vi "Get All Measured Values.vi"(0 "VISA Session In":refnum<visa-resource-name>="OXYMAT", 1 "Target Address":u8=16 format="%.0x", 2 "Source Address":u8=208 format="%.0x", 7 "Use Broadcast?(F)":bool, 11 "error in (no error)":errorcluster) -> (4 "VISA Session Out":refnum<visa-resource-name>, 6 "Message Header":T3 {"Source Address" format="%.0x"; "Target Address" format="%.0x"}, 8 "Measurements":cluster{"Measured value":dbl, "Dimension":T1}[](array[cluster]) {"Measured value" format="%#_6f"}, 10 "Measured variables":T2[](array[typedef]), 13 "Success":bool, 15 "error out":errorcluster)   [LabVIEW 2020, in "Siemens ELAN.lvlib"]
doc: "Using the Siemens ELAN protocol, gets all measured values from a channel. The input boolean 'Use Broadcast?' determines whether the values are actively requested, or whether this VI passively waits for a broadcast telegram. Returns array of measured real values and units of measure, plus a matching array of measured variable types. Also returns a boolean indicating that the addressed device provided a valid response.\n\n$Revision:: 0 $\n$Modtime:: yy-mm-dd hh:mm $\n$Author:: Dboyd $"
uses:
  Siemens ELAN.lvlib
  Unit Dimensions.ctl
  Measured variables.ctl
  Message Header.ctl
  Channel Status.ctl
panel:
  in  "Measured variable":T2
  in  "Dimension":T1
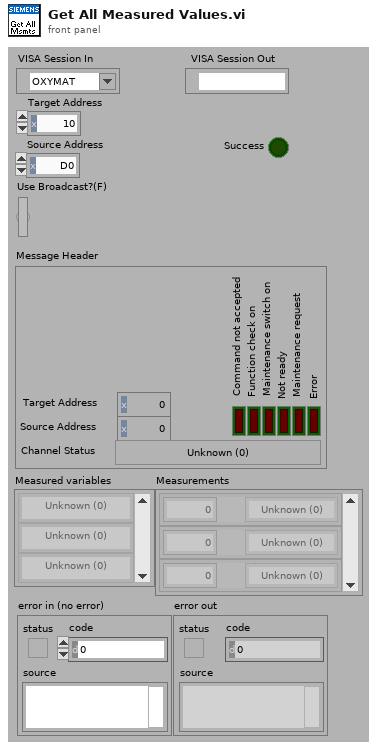
[diagram p1: front panel]
types:
  T1 = typedef "Siemens ELAN.lvlib/Unit Dimensions.ctl" = enum8{"Unknown (0)", "Pure number", "ppm", "ppb", "vpm", "vpm C1", "vpm C3", "vpm C6", "mg C/m^3", "mg/m^3", "%", "% v/v", "% of range", "% saturation", "%/°C", "%/K", "% w/w", "mV/pH", "mV/mbar", "nA/mbar", "S/m", "S/cm", "mS/m", "mS/cm", "uS/m", "uS/cm", "s", "min", "hr", "pA", "mA", "uV", "mV", "V", "mbar", "hPa", "ml/min", "kohm", "MOhm", "S", "°C", "Hz", "pH", "ug/l", "mg/l", "l/min", "uA", "mg/dm^3", "kPa", "kohm*cm", "MOhm*cm", "°", "Unknown (>51)"}
  T2 = typedef "Siemens ELAN.lvlib/Measured variables.ctl" = enum8{"Unknown (0)", "No component", "CO", "CO2", "CH4", "C6H14", "SO2", "NO", "NO2", "CHClF2 (R22)", "C3H8", "C4H10", "O2", "C5H12", "HC", "Pressure", "pH", "Temperature", "C2H4", "C2H2", "C3H6", "C4H6", "C4H8", "C2H6", "NH3", "N2O", "C6H6", "SF6", "CH3OH", "C2H5OH", "CH2Cl2", "C2H4Cl2", "CH3Cl", "C2H4O", "H2O (vapor)", "G/l", "Unknown (36)", "Unknown (37)", "Unknown (38)", "Unknown (39)", "Unknown (40)", "Unknown (41)", "Unknown (42)", "Unknown (43)", "Unknown (44)", "Unknown (45)", "Unknown (46)", "Unknown (47)", "Unknown (48)", "Unknown (49)", "Unknown (50)", "Unknown (51)", "Unknown (52)", "Unknown (53)", "Unknown (54)", "Unknown (55)", "Unknown (56)", "Unknown (57)", "Unknown (58)", "Unknown (59)", "Unknown (60)", "Unknown (61)", "Unknown (62)", "Unknown (63)", "Unknown (64)", "Unknown (65)", "Unknown (66)", "Unknown (67)", "Unknown (68)", "Unknown (69)", "Unknown (70)", "Unknown (71)", "Unknown (72)", "Unknown (73)", "Unknown (74)", "Unknown (75)", "Unknown (76)", "Unknown (77)", "Unknown (78)", "Unknown (79)", "Unknown (80)", "Unknown (81)", "Unknown (82)", "Unknown (83)", "Unknown (84)", "Unknown (85)", "Unknown (86)", "Unknown (87)", "Unknown (88)", "Unknown (89)", "Unknown (90)", "Unknown (91)", "Unknown (92)", "Unknown (93)", "Unknown (94)", "Unknown (95)", "Unknown ((96)", "Unknown (97)", "Unknown (98)", "Unknown (99)", "Ambient Pressure", "Unknown (>100)"}
  T3 = typedef "Siemens ELAN.lvlib/Message Header.ctl" = cluster{"Target Address":u8, "Source Address":u8, "Error":bool, "Maintenance request":bool, "Not ready":bool, "Maintenance switch on":bool, "Function check on":bool, "Command not accepted":bool, "Channel Status":T4}
  T4 = typedef "Siemens ELAN.lvlib/Channel Status.ctl" = enum8{"Unknown (0)", "Warm-up", "Pause", "Standby", "Measure", "Zero calibration", "Adjust component slope", "Unknown (7)", "Adjust curve dip", "Adjust linearization sensitivity", "Adjust temperature compensation", "Adjust pressure compensation", "Adjust linearization zero", "Adjust flow sensor", "Autocal", "Adjust phase", "Zero calibration of O2 sensor", "Synchronous zero calibration", "Purging for synchronous zero calibration", "Adjust analog output", "Adjust analog input", "Cleaning", "Unknown (>21)"}
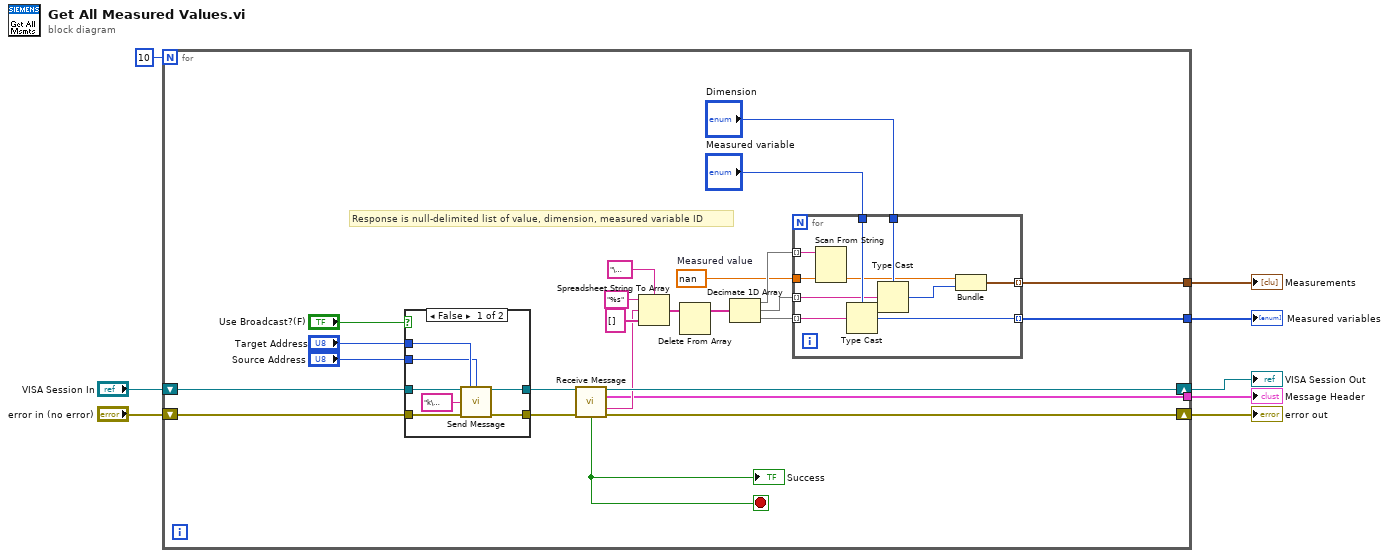
[diagram p0: block diagram]
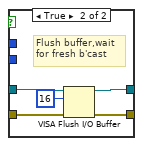
[diagram p2: hidden frame]
diagram:
  n1 = for {
    N: 10 -> [_]
    tunnel: [w13] -> w4
    tunnel: [w12] -> w3
    tunnel: [w11] -> w2
    shift-right: [w29] -> w6
    shift-left: "VISA Session In" -> [w31]
    shift-right: [w28] -> w5
    shift-left: "error in (no error)" -> [w30]
    stop <- w9 stop-if-true
    w14 = nan  # Measured value
    # "Response is null-delimited list of value, dimension, measured variable ID"
    n2 = case shown="False" "Use Broadcast?(F)" {
      tunnel: [w40 w44] -> w33
      tunnel: [w39 w42] -> w32
      tunnel: w31 -> [w38 w45]
      tunnel: w30 -> [w37 w43]
      tunnel: "Target Address" -> [w36 _]
      tunnel: "Source Address" -> [w35 _]
      frame False {
        n3 = call "Send Message.vi"("VISA Session In"=w38, "Target Address"=w36, "Source Address"=w35, "Command"="k\u0002", "error in (no error)"=w37) -> ("VISA Session Out"=w40:refnum<visa-resource-name>, "error out"=w39:errorcluster)  [unwired: 8 in, 1 out]
      }
      frame True {
        # "Flush buffer,wait\nfor fresh b'cast"
        n4 = VISA Flush I/O Buffer(VISA resource name=w45, mask (16)=u16 16, error in (no error)=w43) -> (VISA resource name out=w44:refnum<visa-resource-name>, error out=w42:errorcluster)
      }
    }
    n5 = call "Receive Message.vi"("VISA Session In"=w33, "error in (no error)"=w32) -> ("VISA Session Out"=w29:refnum<visa-resource-name>, "Message Header"=w12:T3, "Response"=w24:string, "Success"=w9:bool, "error out"=w28:errorcluster)  [unwired: 8 in, 1 out]
    "Success" <- w9
    n6 = Spreadsheet String To Array(delimiter (Tab)="\u0000", format string="%s", spreadsheet string=w24, array type (2D Dbl)=string[] []) -> (array=w21:string[])
    n7 = Delete From Array(array=w21) -> (array with subset deleted=w20:string[])  [unwired: 2 in, 1 out]
    n8 = Decimate 1D Array(w20) -> (w15:string[], w18:string[], w19:string[])
    n9 = for {
      tunnel: "Dimension" -> [w55]
      tunnel: w19 -> [w50] mode=indexing
      tunnel: w18 -> [w49] mode=indexing
      tunnel: "Measured variable" -> [w54]
      tunnel: [w53] -> w13 mode=indexing
      tunnel: w15 -> [w52] mode=indexing
      tunnel: w14 -> [w51]
      tunnel: [w46] -> w11 mode=indexing
      n10 = Scan From String(input string=w52, default 1=w51) -> (output 1=w48:dbl)  [unwired: 3 in, 3 out]
      n11 = Type Cast(type=w54, x=w50) -> (*(type *) &x=w53:T2)
      n12 = Type Cast(type=w55, x=w49) -> (*(type *) &x=w47:T1)
      n13 = Bundle("Measured value"=w48, "Dimension"=w47) -> (w46:cluster{"Measured value":dbl, "Dimension":T1})  [unwired: 1 in]
    }
  }
  "VISA Session Out" <- w6
  "error out" <- w5
  "Measured variables" <- w4
  "Message Header" <- w3
  "Measurements" <- w2
